vi "Obtain Buffer.vi"(7 "Buffer Size (10k)":i32=10000 format="%.0p", 8 "error in (no error)":errorcluster, 10 "Create (F)":bool) -> (0 "error out":errorcluster, 3 "Table Queue":refnum<queue>)   [LabVIEW 2025, in "CAN-LIN Raw Bus Capture UI.lvlib"]
uses:
  CAN-LIN Raw Bus Capture UI.lvlib
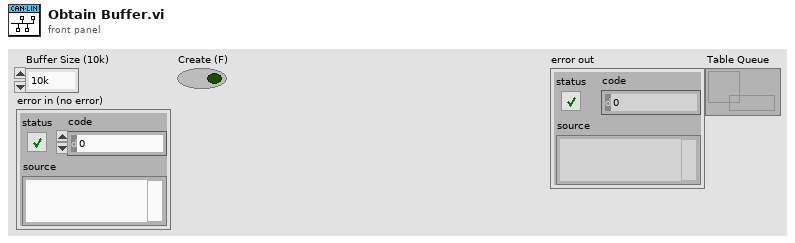
[diagram p1: front panel]
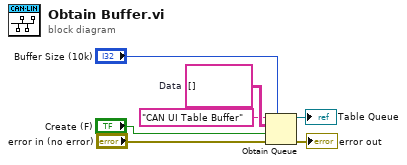
[diagram p0: block diagram]
diagram:
  w3 = string[][] []  # Data
  n1 = Obtain Queue(max queue size (-1, unlimited)="Buffer Size (10k)", name (unnamed)="CAN UI Table Buffer", element data type=w3, create if not found? (T)="Create (F)", error in (no error)="error in (no error)") -> (queue out=→"Table Queue":refnum<queue>, error out=→"error out":errorcluster)  [unwired: 1 out]
